vi "ir.vi"(8 "error in (no error)":errorcluster, 11 "選擇紅外線":enum16{"請選擇紅外線", "紅外線1", "紅外線2", "紅外線3", "紅外線4"}(ring)) -> (0 "error out":errorcluster, 2 "公分":dbl(slide) scale=0.0..200.0)   [LabVIEW 2019]
uses:
  <vilib>/myRIO/Instrument Drivers/Onboard IO/AI/typedefs/AI Reference.ctl
  <vilib>/myRIO/Common/Instrument Driver Framework/Utilities/typedefs/myRIO Generic Hardware Reference.ctl
  <vilib>/myRIO/Common/Instrument Driver Framework/Utilities/typedefs/Hardware Version Enum.ctl
  <vilib>/myRIO/Common/Instrument Driver Framework/Utilities/typedefs/myRIO v1.0 Reference.ctl
  <vilib>/myRIO/Common/Instrument Driver Framework/Utilities/typedefs/Generic FPGA Reference.ctl
  <vilib>/myRIO/Common/Instrument Driver Framework/myRIO v1.0/AI/typedefs/AI Channels List.ctl
  <vilib>/myRIO/Common/Instrument Driver Framework/myRIO v1.0/AI/typedefs/AI Channels Enum.ctl
  <vilib>/myRIO/Common/Instrument Driver Framework/Utilities/typedefs/Analog Scaling Constants List.ctl
  <vilib>/myRIO/Common/Instrument Driver Framework/Utilities/typedefs/Analog Scaling Constants.ctl
  <vilib>/userDefined/High Color/nirio_resource_hc.ctl
  <vilib>/myRIO/Common/Instrument Driver Framework/Utilities/vis/Is FPGA Ref Available.vi
  <vilib>/myRIO/Common/Instrument Driver Framework/myRIO v1.0/AI/vis/myRIO v1.1 Open AI.vi
  <vilib>/myRIO/Instrument Drivers/Onboard IO/AI/vis/Read.vi
  <vilib>/myRIO/Common/Instrument Driver Framework/Utilities/vis/Validate Channels.vi
  <vilib>/myRIO/Common/Instrument Driver Framework/myRIO v1.0/AI/vis/myRIO v1.0 Reserve AI.vi
  <vilib>/myRIO/Common/Instrument Driver Framework/myRIO v1.0/AI/vis/myRIO v1.0 Build MUX Configuration AI.vi
  <vilib>/myRIO/Common/Instrument Driver Framework/myRIO v1.0/Resource Manager/vis/myRIO v1.0 Reserve Channel List.vi
  <vilib>/myRIO/Common/Instrument Driver Framework/myRIO v1.0/Resource Manager/vis/myRIO v1.0 Reserve Channel.vi
  <vilib>/myRIO/Common/Instrument Driver Framework/myRIO v1.0/Resource Manager/vis/myRIO v1.0 Unreserve Channel.vi
  <vilib>/myRIO/Common/Instrument Driver Framework/myRIO v1.0/Resource Manager/vis/myRIO v1.0 Build Mutex Name.vi
  <vilib>/Utility/VariantDataType/GetNumericInfo.vi
  <vilib>/Utility/error.llb/Error Cluster From Error Code.vi
  <vilib>/myRIO/Common/Instrument Driver Framework/myRIO v1.0/myRIO v1.1 Open.vi
  <vilib>/myRIO/Common/Instrument Driver Framework/myRIO v1.0/AI/vis/myRIO v1.0 Get Scaling Constants AI.vi
  <vilib>/myRIO/Common/Instrument Driver Framework/Utilities/vis/IO Manager.vi
  <vilib>/myRIO/Common/Instrument Driver Framework/Utilities/vis/Configuration Manager.vi
  <vilib>/myRIO/Common/Instrument Driver Framework/myRIO v1.0/myRIO v1.0 Close.vi
  <vilib>/myRIO/Common/Instrument Driver Framework/myRIO v1.0/AI/vis/myRIO v1.0 Read AI.vi
  <vilib>/myRIO/Express VI/Onboard IO/AI/AI Express VI.xnode
  <vilib>/myRIO/Instrument Drivers/Onboard IO/AI/vis/myRIO AI Open.xnode
  <vilib>/myRIO/Instrument Drivers/Onboard IO/AI/AI.lvlib
panel:
  out "x*y":dbl
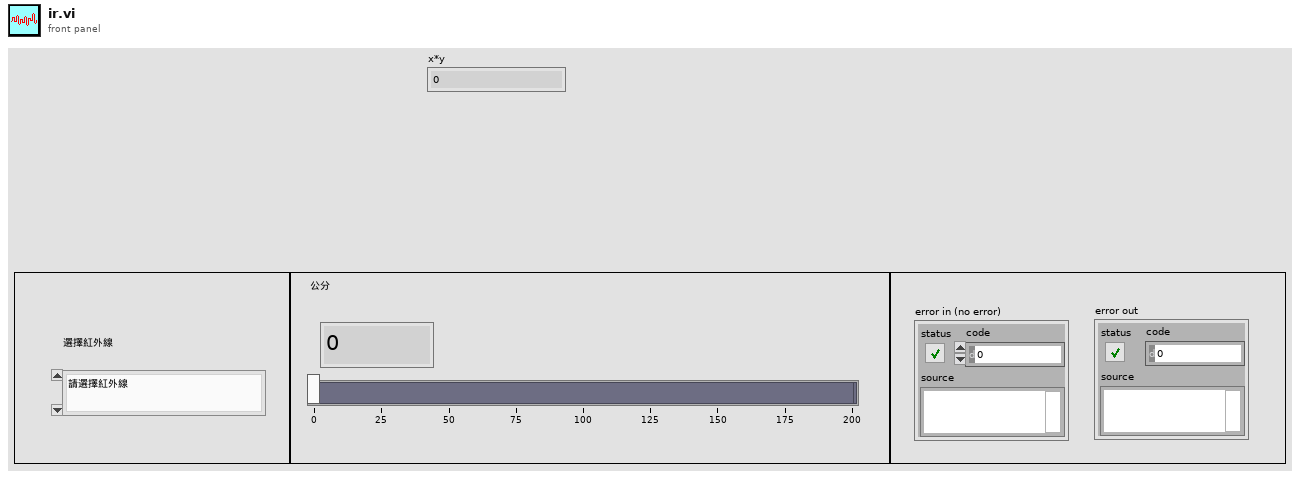
[diagram p1: front panel]
types:
  T1 = typedef "AI.lvlib/AI Reference.ctl" = cluster{"myRIO Reference":T2, "AI Channels List":T6, "AI Scaling Constants List":T8}
  T2 = typedef "myRIO Generic Hardware Reference.ctl" = cluster{"myRIO Model":T3, "myRIO Hardware Reference":T4}
  T3 = typedef "Hardware Version Enum.ctl" = enum16{"Unknown", "myRIO-1900", "myRIO-1950", "roboRIO", "NI ELVIS RIO CM", "ELVIS III"}
  T4 = typedef "myRIO v1.0 Reference.ctl" = cluster{"Generic FPGA Reference":T5, "Allow multiple opens":bool}
  T5 = typedef "Generic FPGA Reference.ctl" = refnum<k20>
  T6 = typedef "AI Channels List.ctl" = T7[]
  T7 = typedef "AI Channels Enum.ctl" = enum16{"Not Connected", "AudioIn/Left", "AudioIn/Right", "C/AI0", "C/AI1", "A/AI0", "A/AI1", "A/AI2", "A/AI3", "A/AI4", "A/AI5", "A/AI6", "A/AI7", "B/AI0", "B/AI1", "B/AI2", "B/AI3", "B/AI4", "B/AI5", "B/AI6", "B/AI7", "AI/AI0", "AI/AI1", "AI/AI2", "AI/AI3", "A/AI0 (DIFF)", "A/AI1 (DIFF)", "A/AI2 (DIFF)", "A/AI3 (DIFF)", "B/AI0 (DIFF)", "B/AI1 (DIFF)", "B/AI2 (DIFF)", "B/AI3 (DIFF)"}
  T8 = typedef "Analog Scaling Constants List.ctl" = T9[]
  T9 = typedef "Analog Scaling Constants.ctl" = cluster{"LSB Weight (Volts)":dbl, "Offset (Volts)":dbl, "Signed?":bool}
  T10 = typedef "nirio_resource_hc.ctl" = tag
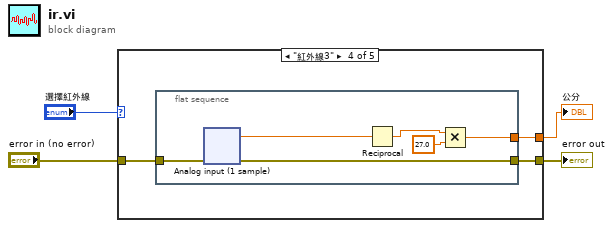
[diagram p0: block diagram]
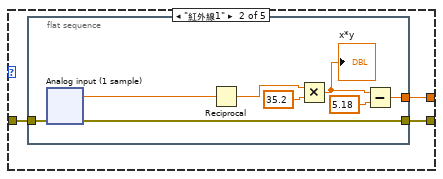
[diagram p3: hidden frame]
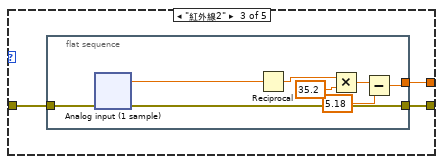
[diagram p4: hidden frame]
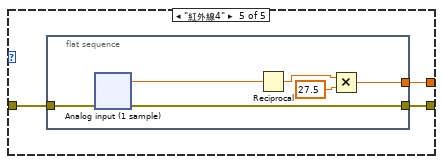
[diagram p5: hidden frame]
diagram:
  n1 = case shown="\"紅外線3\"" "選擇紅外線" {
    tunnel: [w5 w7 w55 w103 w149] -> w3
    tunnel: "error in (no error)" -> [w5 w8 w56 w104 w150]
    tunnel: [_ w6 w54 w102 w148] -> w1
    frame "請選擇紅外線", Default {
    }
    frame "紅外線1" {
      n2 = flat-sequence {
        tunnel: w8 -> [w16]
        tunnel: [w13] -> w7
        tunnel: [w11] -> w6
        frame #0 {
          n3 = xnode "Analog input (1 sample)"("error in (no error)"=w16) -> ("error out"=w13:errorcluster, "A/AI3 (Pin 9)"=w12:dbl)
          n4 = Reciprocal(x=w12) -> (1/x=w15:dbl)
          n5 = Multiply(x=w15, y=35.2) -> (x*y=w9:dbl)
          "x*y" <- w9
          n6 = Subtract(x=w9, y=5.18) -> (x-y=w11:dbl)
        }
      }
    }
    frame "紅外線2" {
      n7 = flat-sequence {
        tunnel: w56 -> [w64]
        tunnel: [w63] -> w55
        tunnel: [w57] -> w54
        frame #0 {
          n8 = xnode "Analog input (1 sample)"("error in (no error)"=w64) -> ("error out"=w63:errorcluster, "A/AI2 (Pin 7)"=w60:dbl)
          n9 = Reciprocal(x=w60) -> (1/x=w62:dbl)
          n10 = Multiply(x=w62, y=35.2) -> (x*y=w59:dbl)
          n11 = Subtract(x=w59, y=5.18) -> (x-y=w57:dbl)
        }
      }
    }
    frame "紅外線3" {
      n12 = flat-sequence {
        tunnel: w104 -> [w110]
        tunnel: [w109] -> w103
        tunnel: [w105] -> w102
        frame #0 {
          n13 = xnode "Analog input (1 sample)"("error in (no error)"=w110) -> ("error out"=w109:errorcluster, "A/AI1 (Pin 5)"=w106:dbl)
          n14 = Reciprocal(x=w106) -> (1/x=w108:dbl)
          n15 = Multiply(x=w108, y=27.0) -> (x*y=w105:dbl)
        }
      }
    }
    frame "紅外線4" {
      n16 = flat-sequence {
        tunnel: w150 -> [w156]
        tunnel: [w151] -> w148
        tunnel: [w155] -> w149
        frame #0 {
          n17 = xnode "Analog input (1 sample)"("error in (no error)"=w156) -> ("error out"=w155:errorcluster, "A/AI0 (Pin 3)"=w152:dbl)
          n18 = Reciprocal(x=w152) -> (1/x=w154:dbl)
          n19 = Multiply(x=w154, y=27.5) -> (x*y=w151:dbl)
        }
      }
    }
  }
  "error out" <- w3
  "公分" <- w1
